vi "draw_P2T.vi"() -> ()   [LabVIEW 2019]
panel:
  out "XY Graph":cluster{dbl[], dbl[]}[](graph)
  in  "He":enum16{"He4", "He3"}(ring)
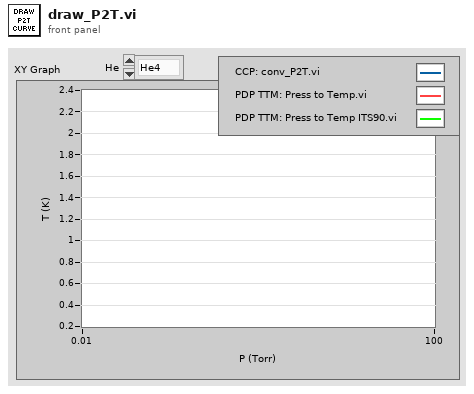
[diagram p1: front panel]
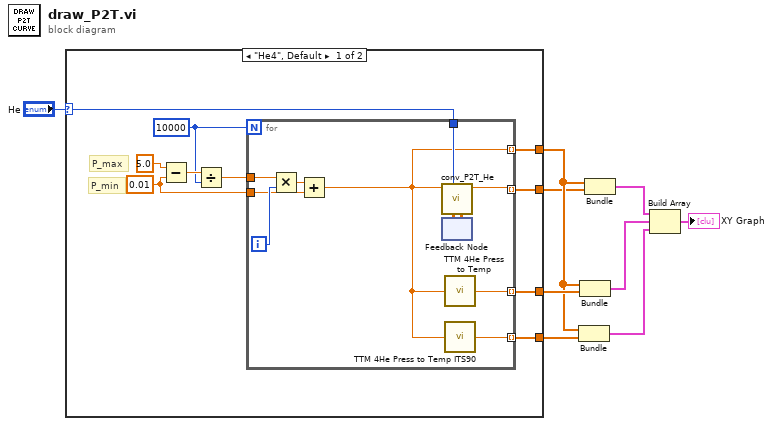
[diagram p0: block diagram]
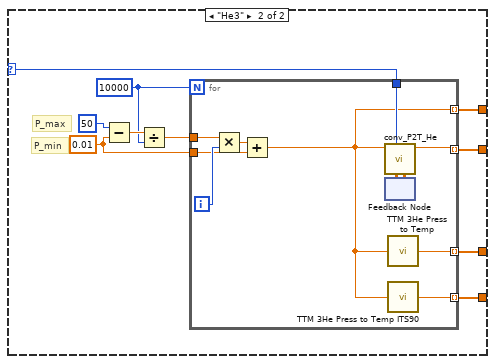
[diagram p2: hidden frame]
diagram:
  n1 = case shown="\"He4\", Default" "He" {
    selector: "He" -> [w19 w35]
    tunnel: [w13 w32] -> w5
    tunnel: [w12 w33] -> w7
    tunnel: [w11 w34] -> w6
    tunnel: [w10 w31] -> w4
    frame "He4", Default {
      w14 = 0.01
      w16 = 10000
      # "P_max"
      # "P_min"
      n2 = Subtract(x=5.0, y=w14) -> (x-y=w17:dbl)
      n3 = Divide(x=w17, y=w16) -> (x/y=w15:dbl)
      n4 = for {
        N: w16 -> [_]
        tunnel: w19 -> [w30]
        tunnel: w15 -> [w29]
        tunnel: w14 -> [w26]
        tunnel: [w21] -> w13 mode=indexing
        tunnel: [w23] -> w10 mode=indexing
        tunnel: [w22] -> w11 mode=indexing
        tunnel: [w20] -> w12 mode=indexing
        i -> [w28]
        n5 = Multiply(x=w29, y=w28) -> (x*y=w27:dbl)
        n6 = Add(x=w27, y=w26) -> (x+y=w21:dbl)
        n7 = feedback #1() -> (w24:dbl[][])  [unwired: 1 in]
        n8 = call "conv_P2T_He.vi"("data_in"=w24, "He"=w30, "P"=w21) -> ("T"=w23:dbl, "data_out"=w25:dbl[][])  [unwired: 6 in, 1 out]
        n9 = feedback-in #1(w25) -> ()
        n10 = call "TTM 4He Press to Temp.vi"("4He Vapor Pressure (torr)"=w21) -> ("4He Temp (K)"=w22:dbl)
        n11 = call "TTM 4He Press to Temp ITS90.vi"("4He Vapor Pressure (torr)"=w21) -> ("4He Temp (K)"=w20:dbl)
      }
    }
    frame "He3" {
      w36 = 0.01
      w38 = 10000
      # "P_max"
      # "P_min"
      n12 = Subtract(x=50, y=w36) -> (x-y=w39:dbl)
      n13 = Divide(x=w39, y=w38) -> (x/y=w37:dbl)
      n14 = for {
        N: w38 -> [_]
        tunnel: w35 -> [w51]
        tunnel: w37 -> [w50]
        tunnel: w36 -> [w47]
        tunnel: [w43] -> w32 mode=indexing
        tunnel: [w44] -> w31 mode=indexing
        tunnel: [w42] -> w34 mode=indexing
        tunnel: [w41] -> w33 mode=indexing
        i -> [w49]
        n15 = Multiply(x=w50, y=w49) -> (x*y=w48:dbl)
        n16 = Add(x=w48, y=w47) -> (x+y=w43:dbl)
        n17 = feedback #2() -> (w45:dbl[][])  [unwired: 1 in]
        n18 = call "conv_P2T_He.vi"("data_in"=w45, "He"=w51, "P"=w43) -> ("T"=w44:dbl, "data_out"=w46:dbl[][])  [unwired: 6 in, 1 out]
        n19 = feedback-in #2(w46) -> ()
        n20 = call "TTM 3He Press to Temp.vi"("3He Vapor pressure in mmhg  between  0.02 and 200."=w43) -> ("corresponding temp K"=w42:dbl)
        n21 = call "TTM 3He Press to Temp ITS90.vi"("3He Vapor Pressure (torr)"=w43) -> ("3He Temp (K)"=w41:dbl)
      }
    }
  }
  n22 = Bundle(w5, w7) -> (w3:cluster{dbl[], dbl[]})  [unwired: 1 in]
  n23 = Bundle(w5, w6) -> (w2:cluster{dbl[], dbl[]})  [unwired: 1 in]
  n24 = Bundle(w5, w4) -> (w1:cluster{dbl[], dbl[]})  [unwired: 1 in]
  n25 = Build Array(w1, w2, w3) -> (→"XY Graph":cluster{dbl[], dbl[]}[])
